vi "LOGNPAGE.vi"() -> ()   [LabVIEW 2018]
panel:
  in  "Tab Control":enum32{"Page 1", "Page 2", "Page 3"}(tab)
  in  "Exit":bool caption="Enter"
  in  "Enter":bool
  in  "Nume":string
  in  "Parola":string
  in  "Login":bool
  in  "Reset":bool
  in  "Close":bool
  in  "Releu":bool caption="Login"
  in  "Temperatura":bool caption="Login"
  in  "Ploaie":bool caption="Login"
  in  "Close 2":bool caption="Login"
  # "Sistem de ajustare ambientala"
  # "De 6VineTancu"
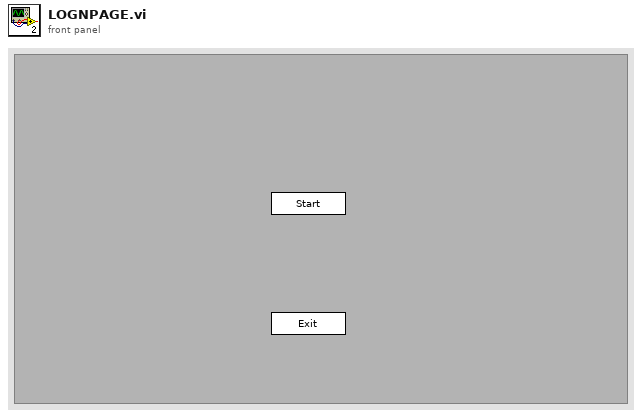
[diagram p1: front panel]
types:
  T1 = enum32{"Invalid", "Standard", "Closed", "Hidden", "Minimized", "Maximized"}
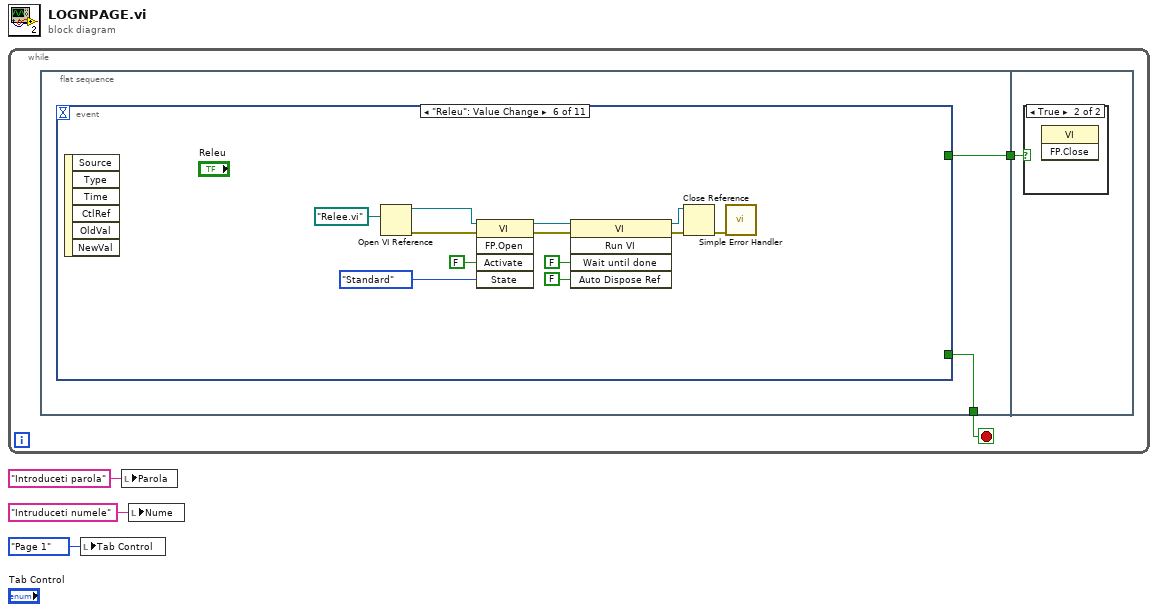
[diagram p0: block diagram]
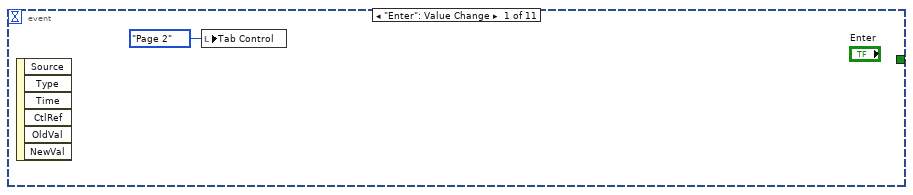
[diagram p2: hidden frame]
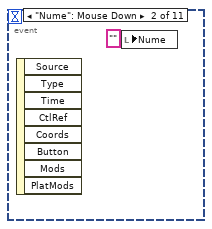
[diagram p3: hidden frame]
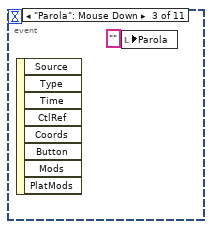
[diagram p4: hidden frame]
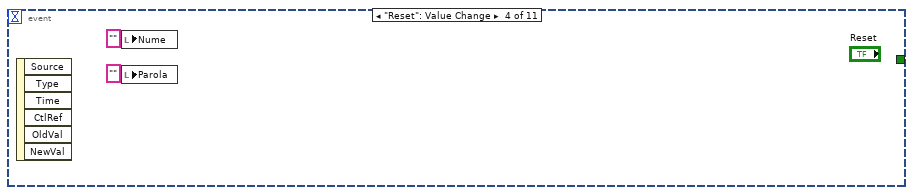
[diagram p5: hidden frame]
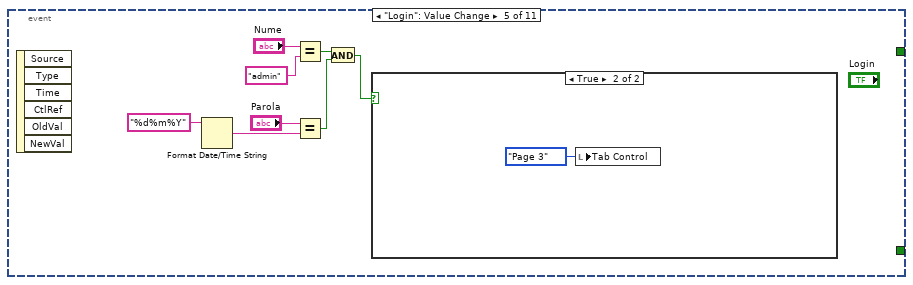
[diagram p6: hidden frame]
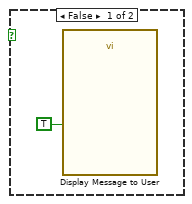
[diagram p7: hidden frame]
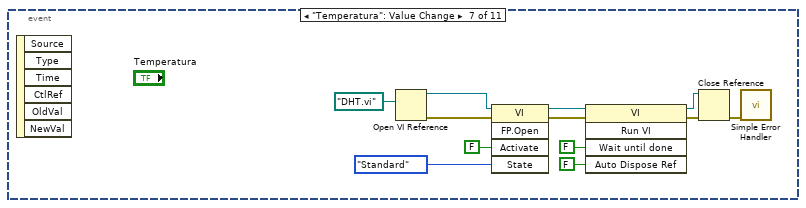
[diagram p8: hidden frame]
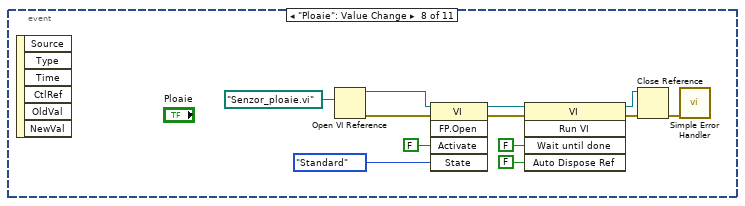
[diagram p9: hidden frame]
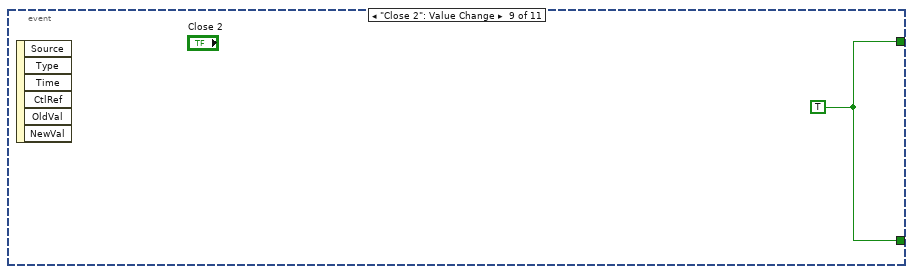
[diagram p10: hidden frame]
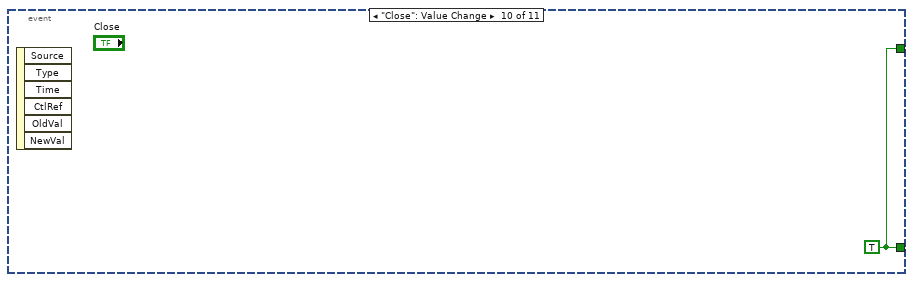
[diagram p11: hidden frame]
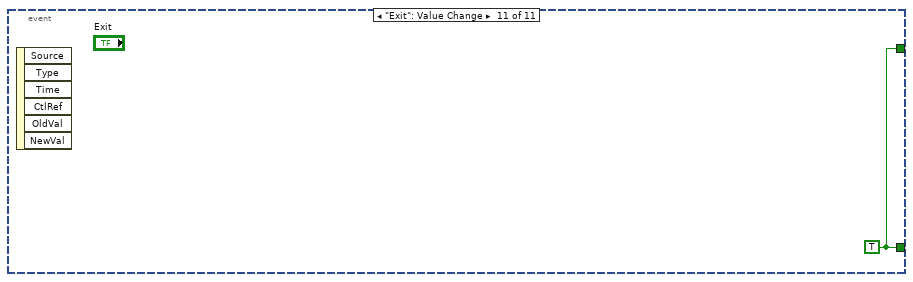
[diagram p12: hidden frame]
diagram:
  n1 = while {
    stop <- w4 stop-if-true
    n2 = flat-sequence {
      tunnel: [w7] -> w5
      tunnel: [w6] -> w4
      tunnel: w5 -> [w62]
      frame #0 {
        n3 = event shown="[5] \"Releu\": Value Change" {
          selector: _ -> [_ _ _ _ _ _ _ _ _ _ _]
          dyn-events: _ -> [_ _ _ _ _ _ _ _ _ _ _]
          timeout: _ -> [_ _ _ _ _ _ _ _ _ _ _]
          tunnel: [_ _ _ _ _ _ _ _ w59 w60 w61] -> w7
          tunnel: [_ _ _ _ _ _ _ _ w59 w60 w61] -> w6
          event "Enter": Value Change {
            n4 = event-data() -> ()  [unwired: 1 in, 6 out]
            n5 = local write "Tab Control"(enum32{"Page 1", "Page 2"}."Page 2" ("Tab Control")) -> ()
          }
          event "Nume": Mouse Down {
            n6 = event-data() -> ()  [unwired: 1 in, 8 out]
            n7 = local write "Nume"("" ("Nume")) -> ()
          }
          event "Parola": Mouse Down {
            n8 = event-data() -> ()  [unwired: 1 in, 8 out]
            n9 = local write "Parola"("" ("Parola")) -> ()
          }
          event "Reset": Value Change {
            n10 = event-data() -> ()  [unwired: 1 in, 6 out]
            n11 = local write "Nume"("" ("Nume")) -> ()
            n12 = local write "Parola"("" ("Parola")) -> ()
          }
          event "Login": Value Change {
            n13 = event-data() -> ()  [unwired: 1 in, 6 out]
            n14 = Format Date/Time String(time format string (%c)="%d%m%Y") -> (date/time string=w16:string)  [unwired: 2 in]
            n15 = Equal?(x="Nume", y="admin") -> (x = y?=w14:bool)
            n16 = Equal?(x="Parola", y=w16) -> (x = y?=w15:bool)
            n17 = And(x=w14, y=w15) -> (x .and. y?=w13:bool)
            n18 = case shown="True" w13 {
              frame False {
                n19 = call "Display Message to User"("Enable"=TRUE) -> ()  [unwired: 9 in, 2 out]
              }
              frame True {
                n20 = local write "Tab Control"(enum32{"Page 1", "Page 2", "Page 3"}."Page 3" ("Tab Control")) -> ()
              }
            }
          }
          event "Releu": Value Change {
            n21 = event-data() -> ()  [unwired: 1 in, 6 out]
            n22 = Open VI Reference(vi path=path "Relee.vi") -> (vi reference=w34:refnum<vi>, error out=w33:errorcluster)  [unwired: 5 in]
            n23 = invoke class="VI" method="FP.Open"(reference=w34, error in=w33, "Activate"=FALSE ("Activate?"), "State"=T1."Standard") -> (reference out=w32:refnum<vi>, error out=w31:errorcluster)  [unwired: 1 in, 3 out]
            n24 = invoke class="VI" method="Run VI"(reference=w32, error in=w31, "Wait until done"=FALSE ("Wait Until Done"), "Auto Dispose Ref"=FALSE ("Auto Dispose Reference")) -> (reference out=w30:refnum<vi>, error out=w29:errorcluster)  [unwired: 1 in, 3 out]
            n25 = Close Reference(reference=w30, error in (no error)=w29) -> (error out=w28:errorcluster)
            n26 = call <vilib>:"Simple Error Handler.vi"("error in (no error)"=w28) -> ()  [unwired: 4 in, 5 out]
          }
          event "Temperatura": Value Change {
            n27 = event-data() -> ()  [unwired: 1 in, 6 out]
            n28 = Open VI Reference(vi path=path "DHT.vi") -> (vi reference=w46:refnum<vi>, error out=w45:errorcluster)  [unwired: 5 in]
            n29 = invoke class="VI" method="FP.Open"(reference=w46, error in=w45, "Activate"=FALSE ("Activate?"), "State"=T1."Standard") -> (reference out=w44:refnum<vi>, error out=w43:errorcluster)  [unwired: 1 in, 3 out]
            n30 = invoke class="VI" method="Run VI"(reference=w44, error in=w43, "Wait until done"=FALSE ("Wait Until Done"), "Auto Dispose Ref"=FALSE ("Auto Dispose Reference")) -> (reference out=w42:refnum<vi>, error out=w41:errorcluster)  [unwired: 1 in, 3 out]
            n31 = Close Reference(reference=w42, error in (no error)=w41) -> (error out=w40:errorcluster)
            n32 = call <vilib>:"Simple Error Handler.vi"("error in (no error)"=w40) -> ()  [unwired: 4 in, 5 out]
          }
          event "Ploaie": Value Change {
            n33 = event-data() -> ()  [unwired: 1 in, 6 out]
            n34 = Open VI Reference(vi path=path "Senzor_ploaie.vi") -> (vi reference=w58:refnum<vi>, error out=w57:errorcluster)  [unwired: 5 in]
            n35 = invoke class="VI" method="FP.Open"(reference=w58, error in=w57, "Activate"=FALSE ("Activate?"), "State"=T1."Standard") -> (reference out=w56:refnum<vi>, error out=w55:errorcluster)  [unwired: 1 in, 3 out]
            n36 = invoke class="VI" method="Run VI"(reference=w56, error in=w55, "Wait until done"=FALSE ("Wait Until Done"), "Auto Dispose Ref"=FALSE ("Auto Dispose Reference")) -> (reference out=w54:refnum<vi>, error out=w53:errorcluster)  [unwired: 1 in, 3 out]
            n37 = Close Reference(reference=w54, error in (no error)=w53) -> (error out=w52:errorcluster)
            n38 = call <vilib>:"Simple Error Handler.vi"("error in (no error)"=w52) -> ()  [unwired: 4 in, 5 out]
          }
          event "Close 2": Value Change {
            w59 = TRUE
            n39 = event-data() -> ()  [unwired: 1 in, 6 out]
          }
          event "Close": Value Change {
            w60 = TRUE
            n40 = event-data() -> ()  [unwired: 1 in, 6 out]
          }
          event "Exit": Value Change {
            w61 = TRUE
            n41 = event-data() -> ()  [unwired: 1 in, 6 out]
          }
        }
      }
      frame #1 {
        n42 = case shown="True" w62 {
          frame False {
          }
          frame True {
            n43 = invoke class="VI" method="FP.Close"() -> ()  [unwired: 3 in, 3 out]
          }
        }
      }
    }
  }
  n44 = local write "Tab Control"(enum32{"Page 1", "Page 2"}."Page 1" ("Tab Control")) -> ()
  n45 = local write "Parola"("Introduceti parola" ("Parola")) -> ()
  n46 = local write "Nume"("Intruduceti numele" ("Nume")) -> ()
